vi "calculate_isope_table.vi"(8 "error in (no error)":errorcluster, 9 "dilution_factor":dbl, 10 "Isotope Table":cluster{"isotope":string, "amount cc":dbl}[](array[cluster])) -> (0 "error out":errorcluster, 2 "Isotope Table new":cluster{"isotope":string, "amount cc":dbl}[](array[cluster]), 5 "PipetteIsotopeTable":cluster{"isotope":string, "amount cc":dbl}[](array[cluster]))   [LabVIEW 2017]
doc: "updates the amount of isotopes in the isotope tabel of the standard b using the dilution factor of the pipette"
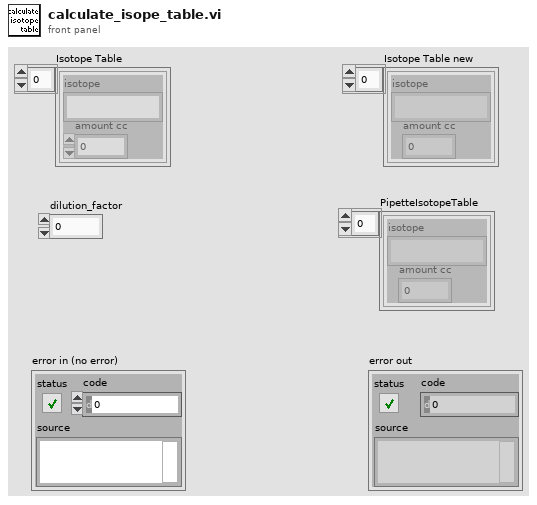
[diagram p1: front panel]
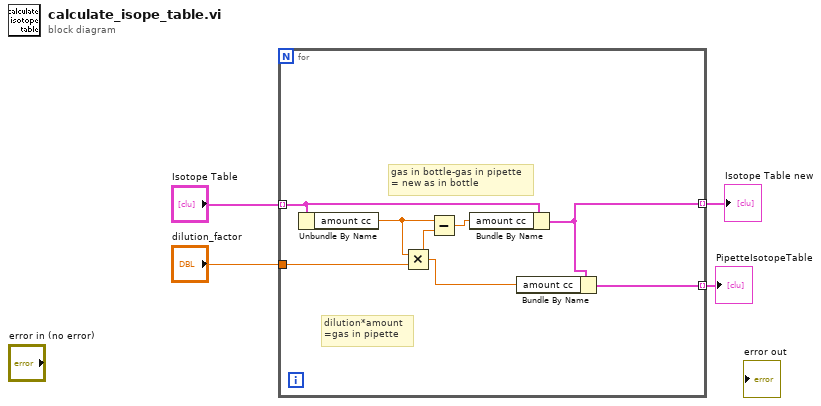
[diagram p0: block diagram]
diagram:
  n1 = for {
    tunnel: "Isotope Table" -> [w8] mode=indexing
    tunnel: "dilution_factor" -> [w10]
    tunnel: [w7] -> w2 mode=indexing
    tunnel: [w5] -> w1 mode=indexing
    # "gas in bottle-gas in pipette\n= new as in bottle"
    # "dilution*amount\n=gas in pipette"
    n2 = Unbundle By Name(w8) -> ("amount cc"=w11:dbl)
    n3 = Multiply(x=w11, y=w10) -> (x*y=w6:dbl)
    n4 = Subtract(x=w11, y=w6) -> (x-y=w9:dbl)
    n5 = Bundle By Name(cluster=w8, "amount cc"=w9) -> (w7:cluster{"isotope":string, "amount cc":dbl})
    n6 = Bundle By Name(cluster=w7, "amount cc"=w6) -> (w5:cluster{"isotope":string, "amount cc":dbl})
  }
  "Isotope Table new" <- w2
  "PipetteIsotopeTable" <- w1
